vi "CompStartTrig.vi"(0 "reference":refnum<k24>, 5 "error in (no error)":errorcluster) -> (7 "TriggerChannel":i32, 8 "DigitalPatternTriggerSense":i32(ring) items=["AbovePattern", "BelowPattern", "EqualPattern", "NotEqualPattern"], 9 "AnalogHWTriggerSense":i32(ring) items=["AboveLevel", "BelowLevel", "RisingEdge", "FallingEdge"], 10 "TriggerChannelStr":string, 11 "ExtTTLTriggerSense":i32(ring) items=["RisingEdge", "FallingEdge"], 12 "Type":i32(ring) items=["None", "ExtTTL", "AnalogHW", "AnalogSW", "DigitalPattern", "Counter"], 13 "AnalogSWTriggerSense":i32(ring) items=["AboveLevel", "BelowLevel", "EqualLevel", "NotEqualLevel", "RisingEdge", "FallingEdge"], 14 "reference out":refnum<k24>, 15 "Level":dbl, 16 "CounterChannelTriggerSense":i32(ring) items=["AboveCount", "BelowCount", "EqualCount", "NotEqualCount", "RisingCount", "FallingCount"], 17 "PretriggerCount":i32, 18 "Variance":dbl, 19 "error out":errorcluster)   [LabVIEW 2009]
uses:
  C:/Program Files/National Instruments/LabVIEW 2009/vi.lib/ULx/ULx_LV.dll
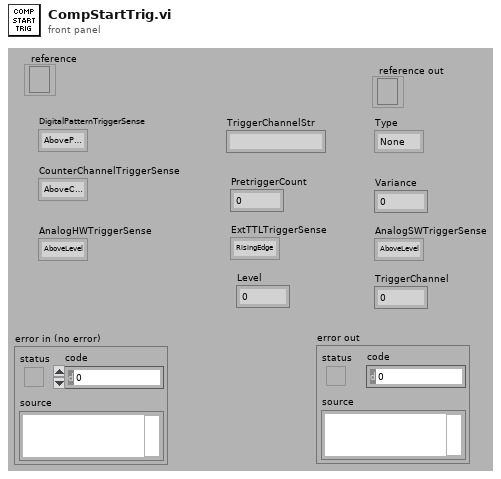
[diagram p1: front panel]
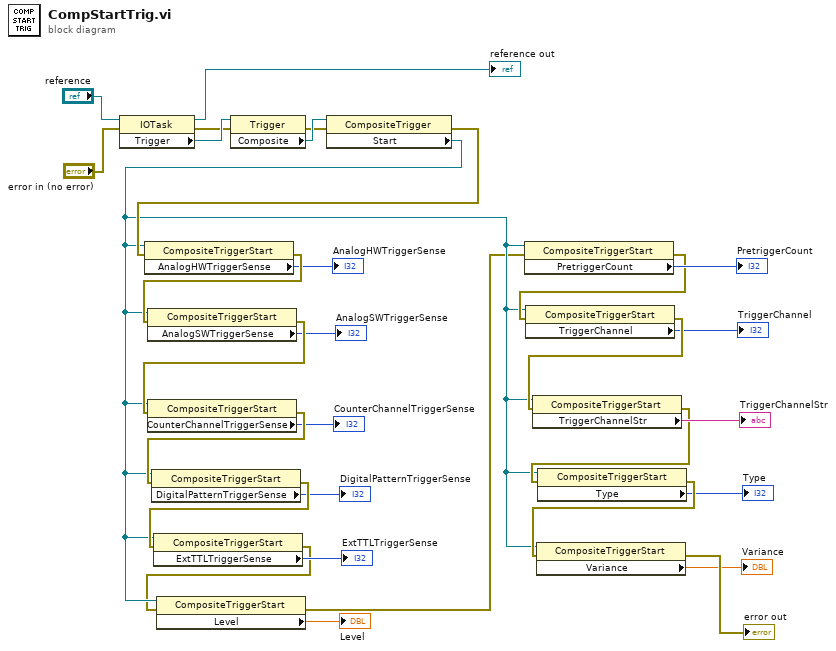
[diagram p0: block diagram]
diagram:
  n1 = property class="IOTask"(reference="reference", error in="error in (no error)") -> (reference out=→"reference out":refnum<k24>, error out=w28:errorcluster, "Trigger"=w31:refnum<k24>)
  n2 = property class="Trigger"(reference=w31, error in=w28) -> (error out=w27:errorcluster, "Composite"=w30:refnum<k24>)  [unwired: 1 out]
  n3 = property class="CompositeTrigger"(reference=w30, error in=w27) -> (error out=w24:errorcluster, "Start"=w4:refnum<k24>)  [unwired: 1 out]
  n4 = property class="CompositeTriggerStart"(reference=w4, error in=w24) -> (error out=w23:errorcluster, "AnalogHWTriggerSense"=→"AnalogHWTriggerSense":i32)  [unwired: 1 out]
  n5 = property class="CompositeTriggerStart"(reference=w4, error in=w23) -> (error out=w22:errorcluster, "AnalogSWTriggerSense"=→"AnalogSWTriggerSense":i32)  [unwired: 1 out]
  n6 = property class="CompositeTriggerStart"(reference=w4, error in=w22) -> (error out=w21:errorcluster, "CounterChannelTriggerSense"=→"CounterChannelTriggerSense":i32)  [unwired: 1 out]
  n7 = property class="CompositeTriggerStart"(reference=w4, error in=w21) -> (error out=w20:errorcluster, "DigitalPatternTriggerSense"=→"DigitalPatternTriggerSense":i32)  [unwired: 1 out]
  n8 = property class="CompositeTriggerStart"(reference=w4, error in=w20) -> (error out=w3:errorcluster, "ExtTTLTriggerSense"=→"ExtTTLTriggerSense":i32)  [unwired: 1 out]
  n9 = property class="CompositeTriggerStart"(reference=w4, error in=w3) -> (error out=w2:errorcluster, "Level"=→"Level":dbl)  [unwired: 1 out]
  n10 = property class="CompositeTriggerStart"(reference=w4, error in=w2) -> (error out=w7:errorcluster, "PretriggerCount"=→"PretriggerCount":i32)  [unwired: 1 out]
  n11 = property class="CompositeTriggerStart"(reference=w4, error in=w7) -> (error out=w6:errorcluster, "TriggerChannel"=→"TriggerChannel":i32)  [unwired: 1 out]
  n12 = property class="CompositeTriggerStart"(reference=w4, error in=w6) -> (error out=w13:errorcluster, "TriggerChannelStr"=→"TriggerChannelStr":string)  [unwired: 1 out]
  n13 = property class="CompositeTriggerStart"(reference=w4, error in=w13) -> (error out=w19:errorcluster, "Type"=→"Type":i32)  [unwired: 1 out]
  n14 = property class="CompositeTriggerStart"(reference=w4, error in=w19) -> (error out=→"error out":errorcluster, "Variance"=→"Variance":dbl)  [unwired: 1 out]
